vi "get supported types.vi"(8 "error in":errorcluster, 11 "Tagbus PID Module configuration in":refnum<class "PID Module configuration.lvclass">) -> (0 "error out":errorcluster, 2 "supported types":T1[](array[typedef]), 3 "Tagbus PID Module configuration out":refnum<class "PID Module configuration.lvclass">)   [LabVIEW 2014, in "PID Module configuration.lvclass"]
doc: "Provides an interface for determining the targets supported by a given configuration/runtime class pairing. This should be overridden by any useful child class."
uses:
  PID Module configuration.lvclass
  <vilib>/NI/Tag Bus/tag/Data Type.ctl
  <vilib>/NI/Tag Bus/tag/tag descriptor.lvclass
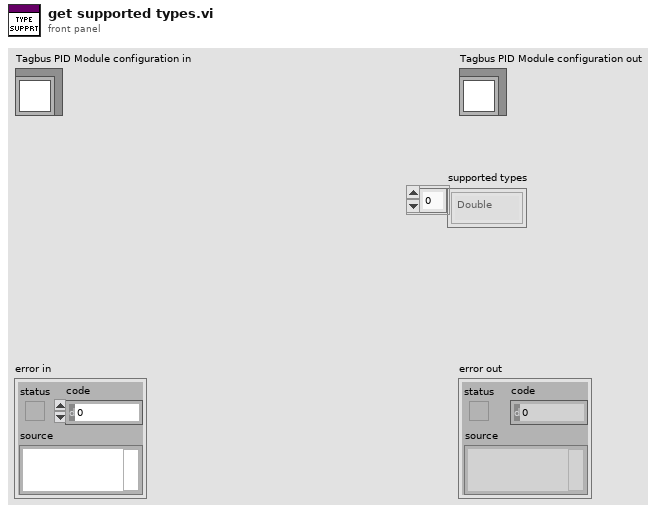
[diagram p1: front panel]
types:
  T1 = typedef "tag bus.lvlib/tag descriptor.lvclass/Data Type.ctl" = enum16{"Double", "Single", "I64", "I32", "I16", "I8", "U64", "U32", "U16", "U8", "Boolean", "String", "Array of Double", "Array of Single", "Array of I64", "Array of I32", "Array of I16", "Array of I8", "Array of U64", "Array of U32", "Array of U16", "Array of U8", "Array of Boolean", "Array of String"}
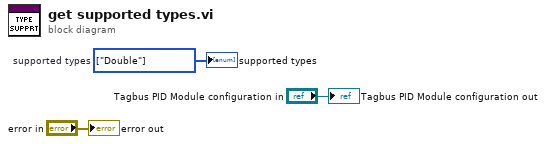
[diagram p0: block diagram]
diagram:
  w1 = T1[] [enum."Double"] items=["Double", "Single", "I64", "I32", "I16", "I8", "U64", "U32", "U16", "U8", "Boolean", "String", "Array of Double", "Array of Single", "Array of I64", "Array of I32", "Array of I16", "Array of I8", "Array of U64", "Array of U32", "Array of U16", "Array of U8", "Array of Boolean", "Array of String"]  # supported types
  "error out" <- "error in"
  "Tagbus PID Module configuration out" <- "Tagbus PID Module configuration in"
  "supported types" <- w1
